vi "Merge Errors from Array.vi"(8 "Error Array In":errorcluster[](array[cluster])) -> (0 "error out":errorcluster)   [LabVIEW 2016, in "PXImc Router.lvlib"]
uses:
  PXImc Router.lvlib
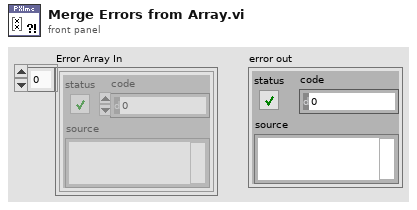
[diagram p1: front panel]
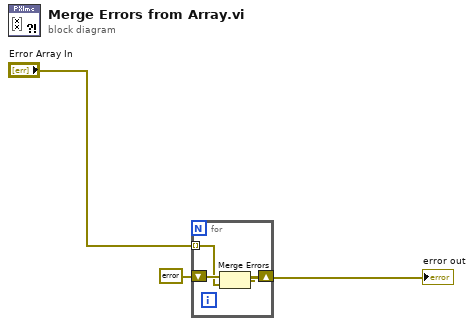
[diagram p0: block diagram]
diagram:
  n1 = for {
    tunnel: "Error Array In" -> [w5] mode=indexing
    shift-right: [w4] -> w3
    shift-left: errorcluster {"status"=FALSE, "code"=0, "source"=""} ("error constant") -> [w6]
    n2 = Merge Errors(w6, w5) -> (w4:errorcluster)
  }
  "error out" <- w3
